vi "PrefixAdder.vi"(0 "No prefix":dbl) -> (1 "Nano":dbl, 2 "Pico":dbl, 3 "Femto":dbl, 4 "Atto":dbl)   [LabVIEW 2019]
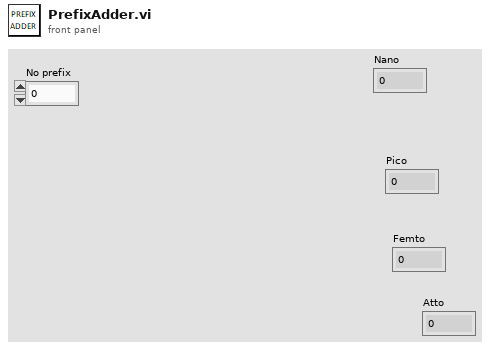
[diagram p1: front panel]
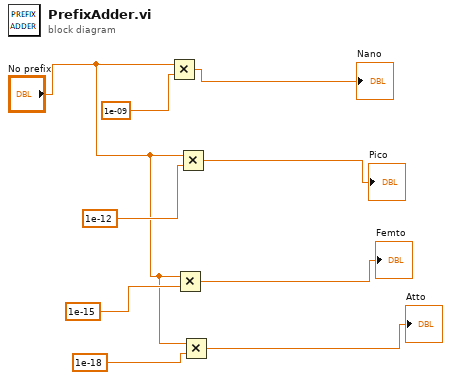
[diagram p0: block diagram]
diagram:
  n1 = Multiply(x="No prefix", y=1e-09) -> (x*y=→"Nano":dbl)
  n2 = Multiply(x="No prefix", y=1e-15) -> (x*y=→"Femto":dbl)
  n3 = Multiply(x="No prefix", y=1e-12) -> (x*y=→"Pico":dbl)
  n4 = Multiply(x="No prefix", y=1e-18) -> (x*y=→"Atto":dbl)
